vi "ARM_DASH_WRITE.vi"   [LabVIEW 2023]
uses:
  ARM_GLOBALS.vi
  <vilib>/Rock Robotics/Network Tables/NT Write Boolean.vi
  <vilib>/Rock Robotics/Network Tables/NT Write Number.vi
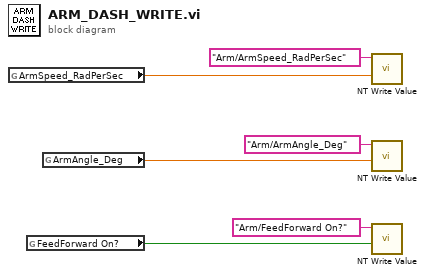
[diagram p0: block diagram]
diagram:
  n1 = global read "ARM_GLOBALS.vi" "ArmSpeed_RadPerSec"() -> (w3:dbl)
  n2 = global read "ARM_GLOBALS.vi" "FeedForward On?"() -> (w1:bool)
  n3 = global read "ARM_GLOBALS.vi" "ArmAngle_Deg"() -> (w4:dbl)
  n4 = call-poly <vilib>:"NT Write Value.vi"("value"=w3, "name"="Arm/ArmSpeed_RadPerSec") -> ()  [unwired: 9 in, 1 out]
  n5 = call-poly <vilib>:"NT Write Value.vi"("value"=w4, "name"="Arm/ArmAngle_Deg") -> ()  [unwired: 9 in, 1 out]
  n6 = call-poly <vilib>:"NT Write Value.vi"("value"=w1, "name"="Arm/FeedForward On?") -> ()  [unwired: 9 in, 1 out]
